vi "Set Panel Level.vi"(6 "Mouse Position":T1, 7 "User VI Ref":refnum<vi>, 8 "Is Multi-select?":bool, 9 "Remaining Items":refnum<vi>[](array[refnum]), 10 "Affected Items":T8, 11 "Menu Refnum":refnum<k9>) -> (3 "Menu Items To Add":T2[](array[typedef]))   [LabVIEW 2021]
doc: "This implementation of the right click menu VI will set the \"UI Theme Level\" for a given control(s) for a VI. It will categorize the type of the control style that is being used so that Theme-ing can be applied appropriately.\n\n<b>Original</b>: This VI is part of a plug-in for modifying the LabVIEW shortcut menus. This is the builder VI which is called when the shortcut menu is built. It tells LabVIEW which shortcut menu items to add to the menu."
uses:
  <resource>/plugins/PopupMenus/support/Shortcut Menu Item Definition.ctl
  <resource>/plugins/PopupMenus/support/Transaction Control.ctl
  <resource>/plugins/PopupMenus/support/Position In Menu.ctl
  <resource>/plugins/PopupMenus/support/Relative Position.ctl
  <resource>/plugins/PopupMenus/support/Checkmark Status.ctl
  <resource>/plugins/PopupMenus/support/Enabled Menu Item Status.ctl
  Set Panel Level.ctl
  <vilib>/Utility/miscctls.llb/LVPositionTypeDef.ctl
  4ff4612b-3443-4282-827c-392bf86662e1.vi
  Material SubVIs/Material SubVIs.lvlib
panel:
  # "Rules a popup plug-in must follow:\n* This VI's file name must match the file name of the LLB -- only the file extensions should be different.\n* This VI must have debugging disabled or it will be ignored as a plug-in.\n* For all menu items, \"tag suffix + file name of this VI\" must be less than 240 characters.\n* You can disconnect the \"Affected Items\" from the typedef to make the plug-in load faster. The typedef is only there to assist you in keeping this VI and the execution VI using to the same type.\n* All controls on this panel except \"Affected Items\" are locked to prevent accidental edits. Do not change the types or the names of controls other than the elements inside the \"Affected Items\" cluster.\n* See Context Help for more information on the individual controls."
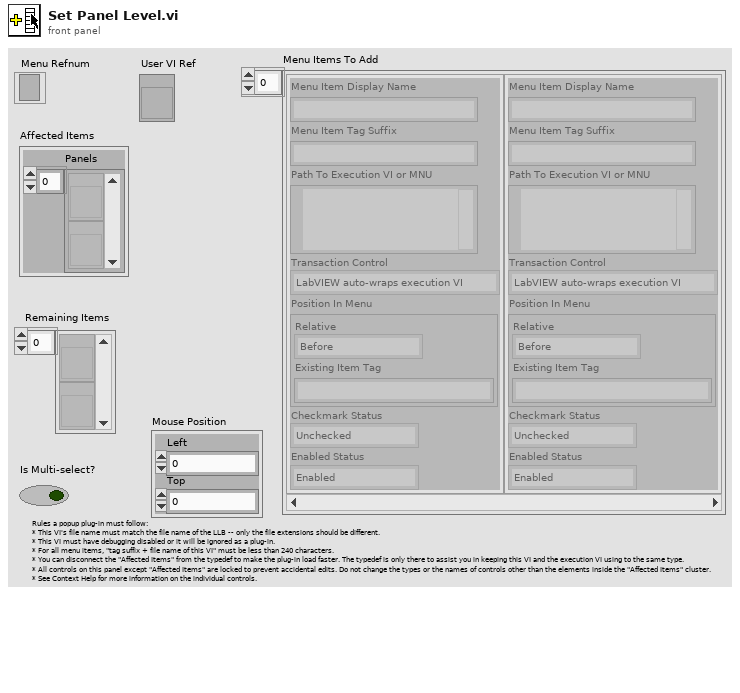
[diagram p1: front panel]
types:
  T1 = typedef "LVPositionTypeDef.ctl" = cluster{"Left":i32, "Top":i32}
  T2 = typedef "Shortcut Menu Item Definition.ctl" = cluster{"Menu Item Display Name":string, "Menu Item Tag Suffix":string, "Path To Execution VI or MNU":path, "Transaction Control":T3, "Position In Menu":T4, "Checkmark Status":T6, "Enabled Status":T7}
  T3 = typedef "Transaction Control.ctl" = enum8{"LabVIEW auto-wraps execution VI", "Execution VI will define if needed"}
  T4 = typedef "Position In Menu.ctl" = cluster{"Relative":T5, "Existing Item Tag":string}
  T5 = typedef "Relative Position.ctl" = enum8{"Before", "Instead of", "After", "Into Submenu"}
  T6 = typedef "Checkmark Status.ctl" = enum8{"Unchecked", "Checked"}
  T7 = typedef "Enabled Menu Item Status.ctl" = enum8{"Enabled", "Disabled"}
  T8 = typedef "Set Panel Level.ctl" = cluster{"Panels":refnum<vi>[]}
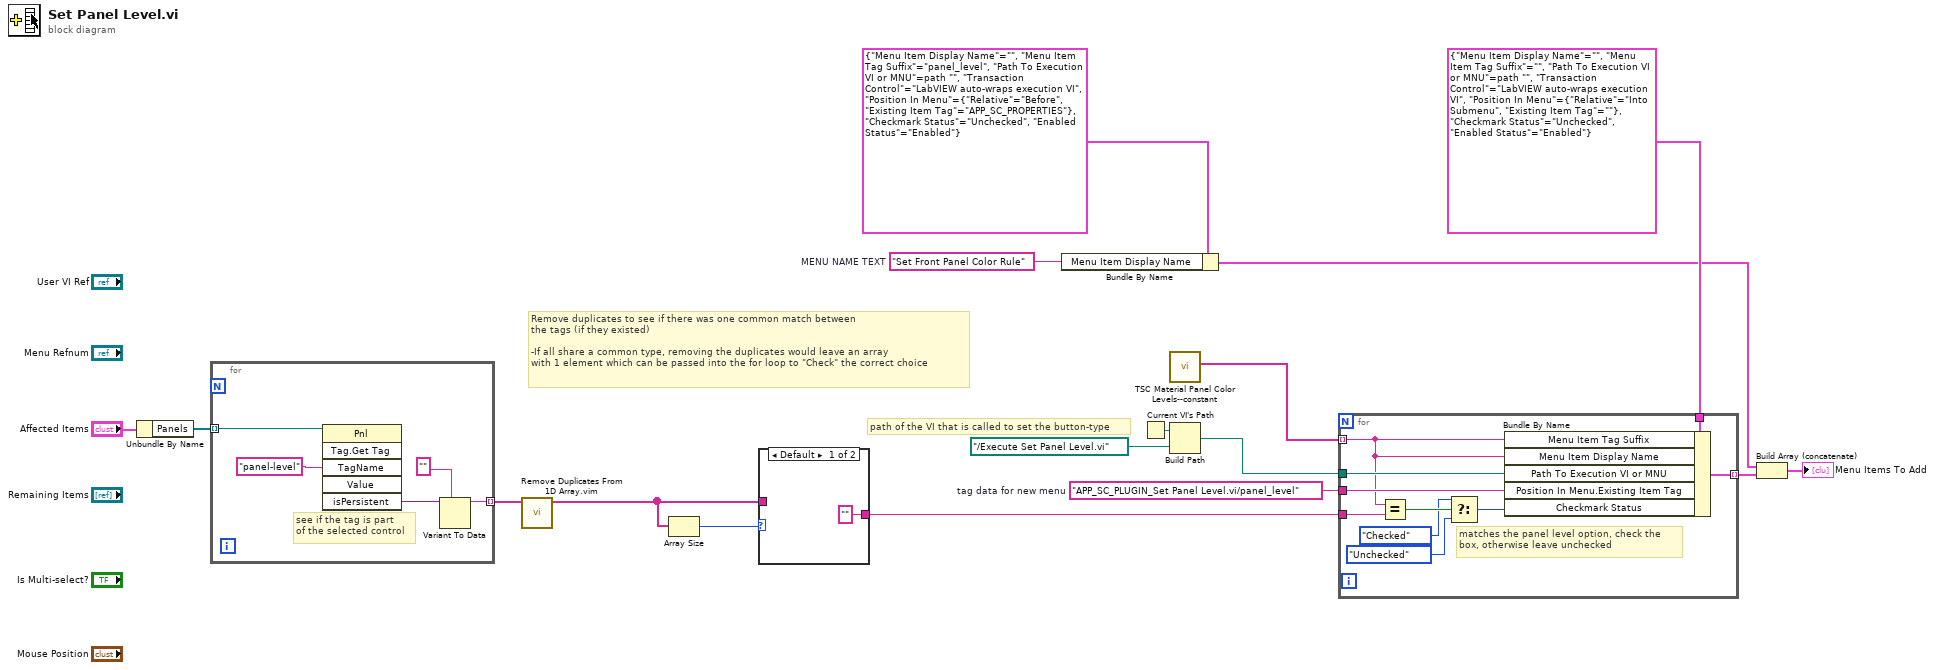
[diagram p0: block diagram]
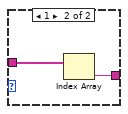
[diagram p2: hidden frame]
diagram:
  w1 = "APP_SC_PLUGIN_Set Panel Level.vi/panel_level"  # tag data for new menu
  w2 = "Set Front Panel Color Rule"  # MENU NAME TEXT
  # "Remove duplicates to see if there was one common match between\nthe tags (if they existed)\n\n-If all share a common type, removing the duplicates would leave an array\nwith 1 element which can be passed into the for loop to \"Check\" the correct choice"
  # "path of the VI that is called to set the button-type"
  n1 = Unbundle By Name("Affected Items") -> ("Panels"=w13:refnum<vi>[])
  n2 = for {
    tunnel: w13 -> [w18] mode=indexing
    tunnel: [w19] -> w10 mode=indexing
    # "see if the tag is part \nof the selected control"
    n3 = invoke class="Pnl" method="Tag.Get Tag"(reference=w18, "TagName"="panel-level" ("Tag Name")) -> ("isPersistent"=w21:variant)  [unwired: 4 in, 5 out]
    n4 = Variant To Data(type="", Variant=w21) -> (data=w19:string)  [unwired: 1 in, 1 out]
  }
  n5 = call "Remove Duplicates From 1D Array.vim"("array"=w10) -> ("array with duplicates removed"=w11:string[])  [unwired: 10 in]
  n6 = Array Size(array=w11) -> (size(s)=w12:i32)
  n7 = case shown="Default" w12 {
    tunnel: w11 -> [_ w25]
    tunnel: ["" w24] -> w9
    frame Default {
    }
    frame 1 {
      n8 = Index Array(array=w25) -> (element=w24:string)  [unwired: 1 in]
    }
  }
  n9 = Bundle By Name(cluster=T2 {"Menu Item Display Name"="", "Menu Item Tag Suffix"="panel_level", "Path To Execution VI or MNU"=path "", "Transaction Control"=enum."LabVIEW auto-wraps execution VI", "Position In Menu"={"Relative"=enum."Before", "Existing Item Tag"="APP_SC_PROPERTIES"}, "Checkmark Status"=enum."Unchecked", "Enabled Status"=enum."Enabled"} ("Cluster"), "Menu Item Display Name"=w2) -> (w5:T2)
  n10 = Current VI's Path() -> (path=w16:path)
  n11 = call "TSC Material Panel Color Levels--constant.vi"() -> ("front panel color levels"=w8:string[])  [unwired: 11 in]
  n12 = Build Path(base path=w16, name or relative path=path "../Execute Set Panel Level.vi" ("execute path")) -> (appended path=w3:path)
  n13 = for {
    tunnel: T2 {"Menu Item Display Name"="", "Menu Item Tag Suffix"="", "Path To Execution VI or MNU"=path "", "Transaction Control"=enum."LabVIEW auto-wraps execution VI", "Position In Menu"={"Relative"=enum."Into Submenu", "Existing Item Tag"=""}, "Checkmark Status"=enum."Unchecked", "Enabled Status"=enum."Enabled"} ("Cluster") -> [w35]
    tunnel: [w34] -> w4 mode=indexing
    tunnel: w3 -> [w33]
    tunnel: w1 -> [w32]
    tunnel: w8 -> [w26] mode=indexing
    tunnel: w9 -> [w28]
    # "matches the panel level option, check the \nbox, otherwise leave unchecked"
    n14 = Equal?(x=w26, y=w28) -> (x = y?=w31:bool)
    n15 = Select(t=Checkmark_Status."Checked" ("Checkmark Status"), s=w31, f=Checkmark_Status."Unchecked" ("Checkmark Status")) -> (s? t:f=w27:T6)
    n16 = Bundle By Name(cluster=w35, "Menu Item Tag Suffix"=w26, "Menu Item Display Name"=w26, "Path To Execution VI or MNU"=w33, "Position In Menu.Existing Item Tag"=w32, "Checkmark Status"=w27) -> (w34:T2)
  }
  n17 = Build Array (concatenate)(w5, w4) -> (→"Menu Items To Add":T2[])
